vi "Ping.vi"() -> ()   [LabVIEW 2020]
panel:
  in  "Stop":bool
  out "Memory Usage History":sgl(graph)
  out "Memory Usage":sgl
  out "error out":errorcluster
  in  "stop":bool
  out "CPU Usage (%)":sgl(slide) scale=0.0..100.0
  out "Processor History":sgl(graph)
  out "cpu usage":sgl
  out "System Status":string
  in  "STOP VI":bool
  in  "PING IP":bool
  out "IP Free?":bool
  in  "IP Address to Ping":string="0.0.0.0"
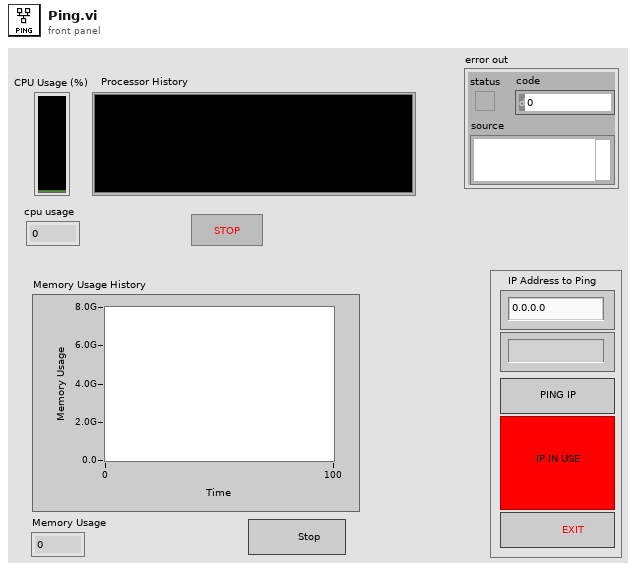
[diagram p1: front panel]
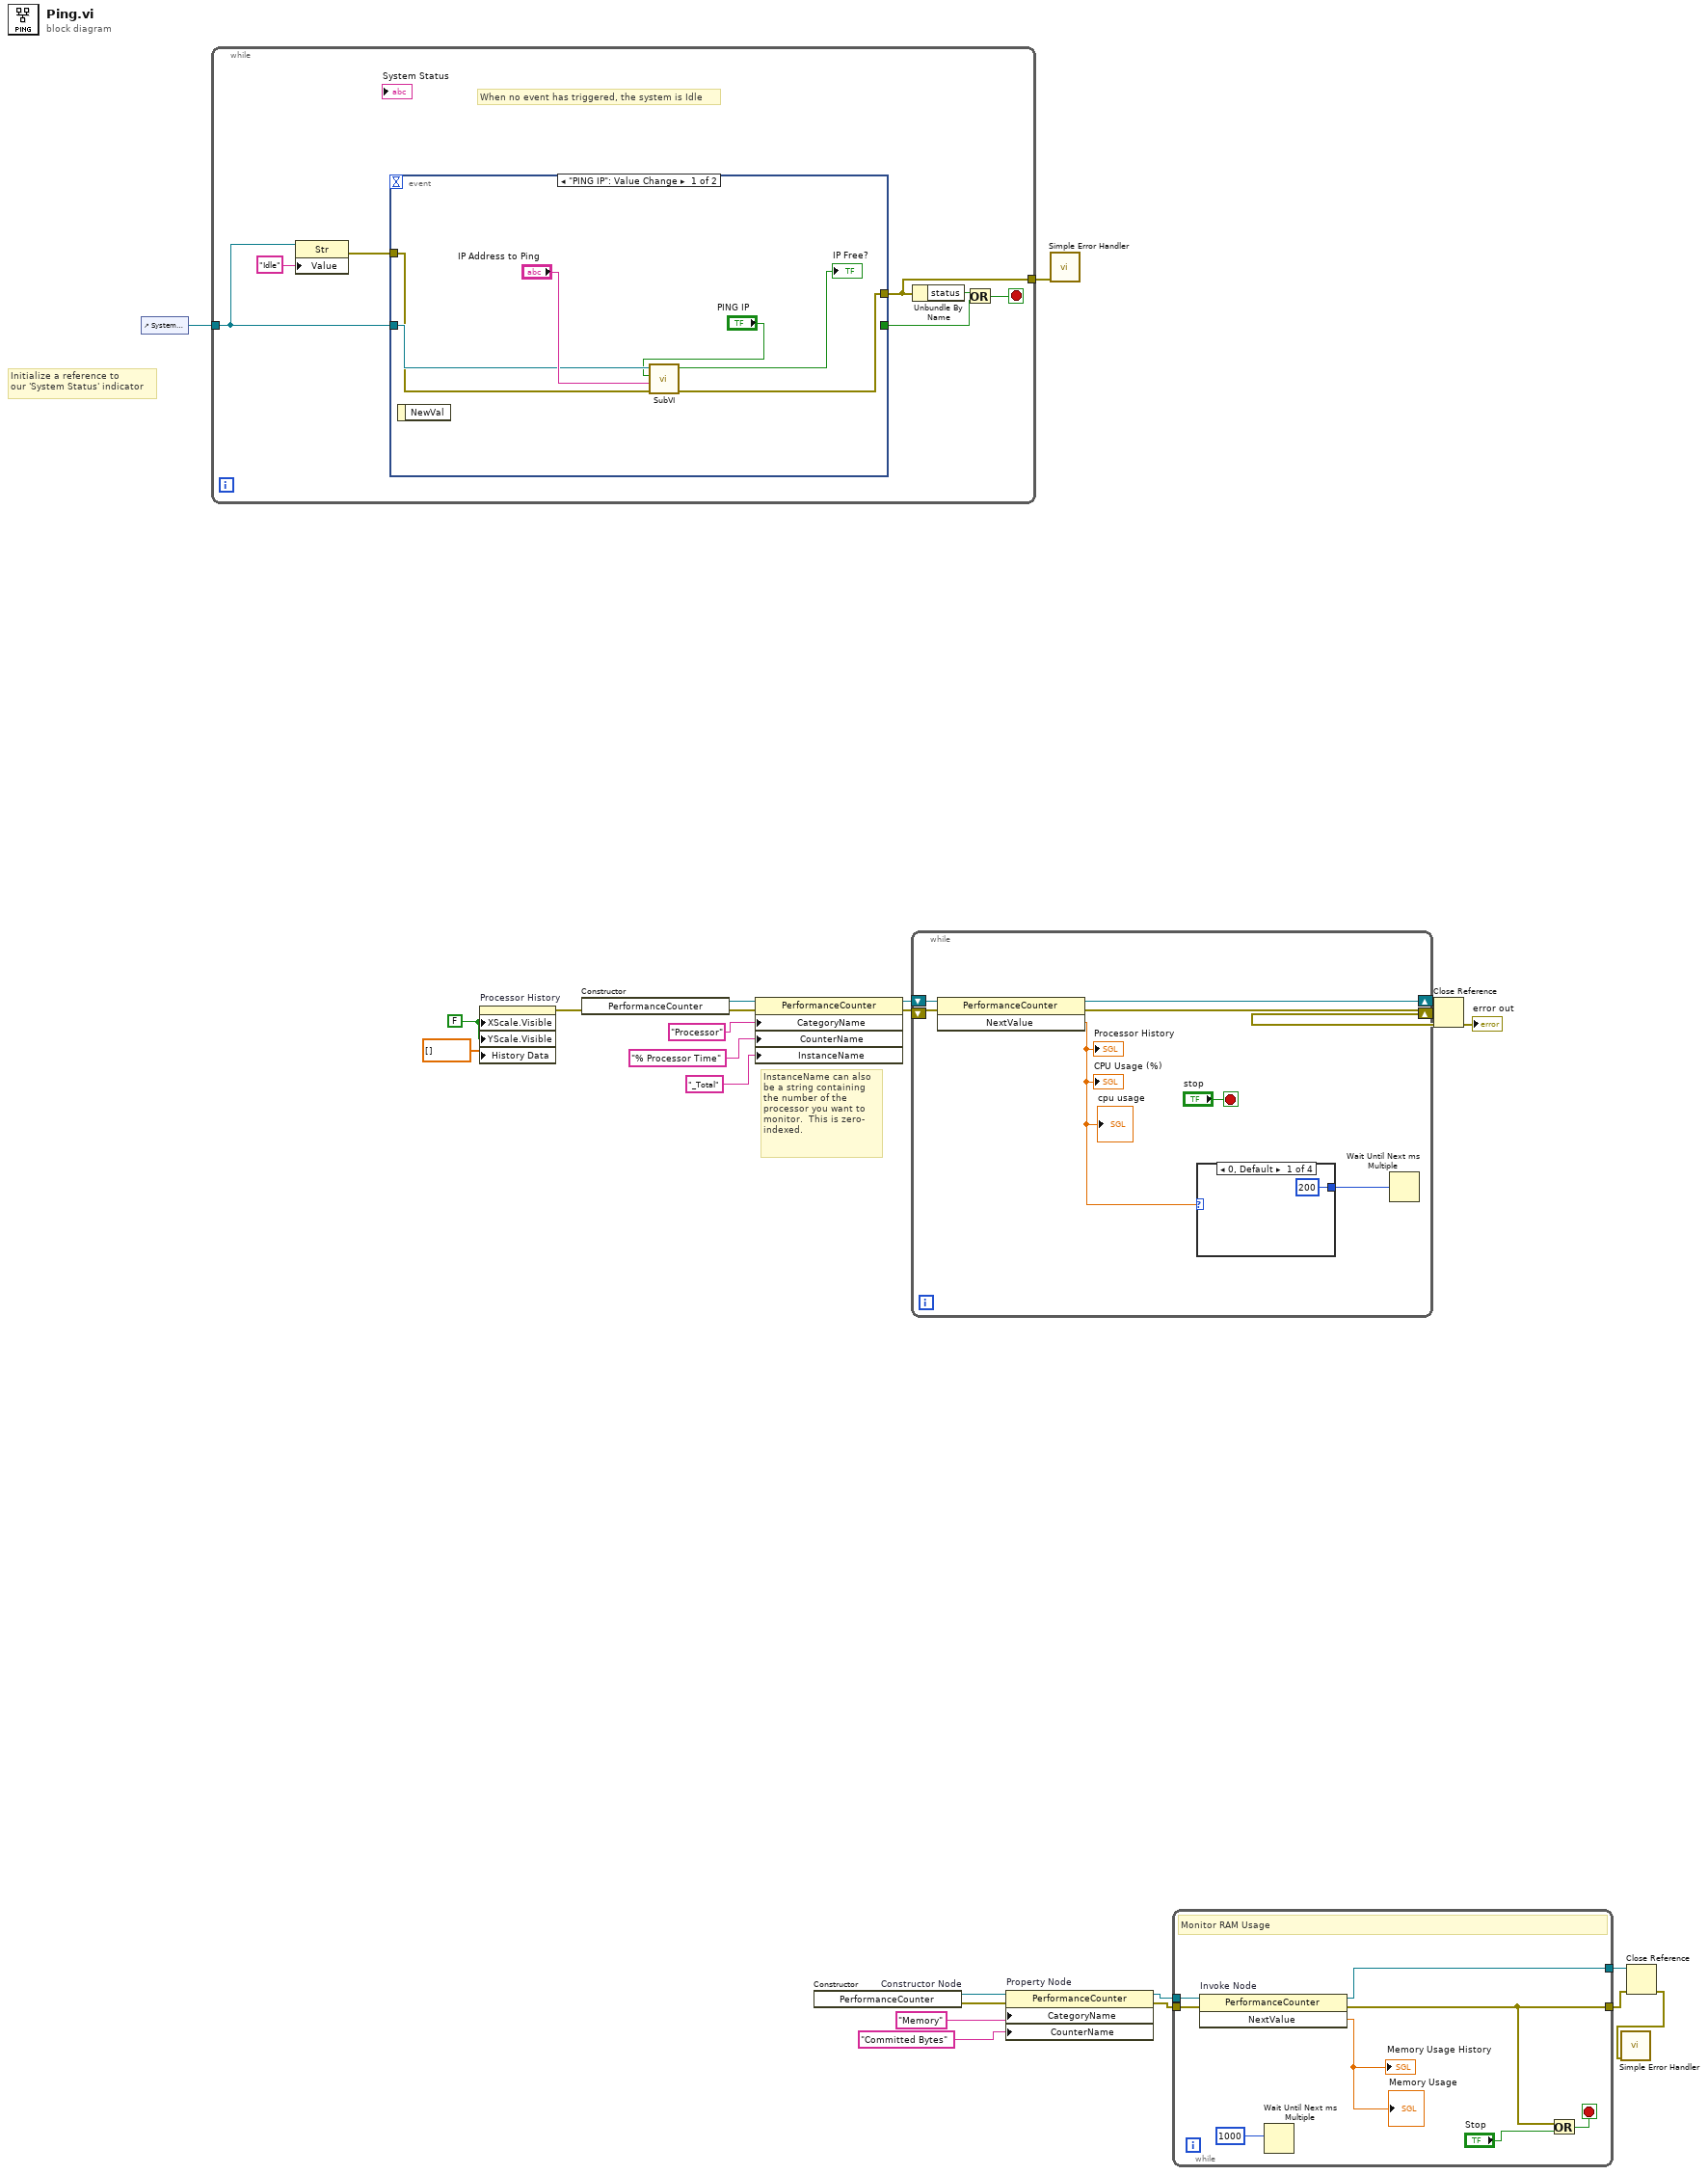
[diagram p0: block diagram]
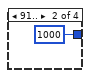
[diagram p2: hidden frame]
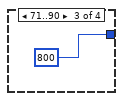
[diagram p3: hidden frame]
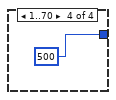
[diagram p4: hidden frame]
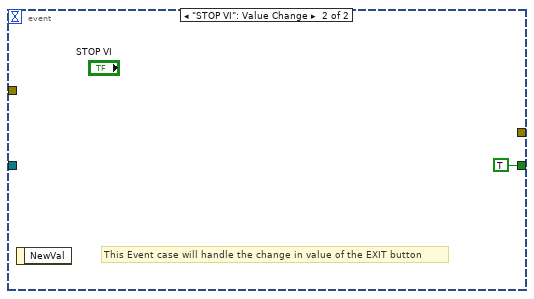
[diagram p5: hidden frame]
diagram:
  w13 = FALSE ("X Scale.Visible")
  # "InstanceName can also\nbe a string containing\nthe number of the\nprocessor you want to\nmonitor.  This is zero-\nindexed."
  # "Initialize a reference to\nour 'System Status' indicator"
  n1 = control-ref of="System Status"() -> (w23:refnum<vi>)
  n2 = while {
    tunnel: [w31] -> w24
    tunnel: w23 -> [w27]
    stop <- w26 stop-if-true
    # "When no event has triggered, the system is Idle"
    n3 = property class="Str"(reference=w27, "Value"="Idle" ("System Status")) -> (error out=w25:errorcluster)  [unwired: 1 in, 1 out]
    n4 = event shown="[0] \"PING IP\": Value Change" {
      selector: _ -> [_ _]
      dyn-events: _ -> [_ _]
      timeout: _ -> [_ _]
      tunnel: [w37 _] -> w31
      tunnel: [_ TRUE] -> w29
      tunnel: w27 -> [w35 _]
      tunnel: w25 -> [w34 _]
      event "PING IP": Value Change {
        n5 = event-data() -> ()  [unwired: 1 in, 1 out]
        n6 = call "SubVI.vi"("error in (no error)"=w34, "IP Address to Ping"="IP Address to Ping", "PING IP"="PING IP", "String in"=w35) -> ("error out"=w37:errorcluster, "IP Free?"=→"IP Free?":bool)  [unwired: 6 in]
      }
      event "STOP VI": Value Change {
        # "This Event case will handle the change in value of the EXIT button"
        n7 = event-data() -> ()  [unwired: 1 in, 1 out]
      }
    }
    n8 = Unbundle By Name(w31) -> ("status"=w30:bool)
    n9 = Or(x=w30, y=w29) -> (x .or. y?=w26:bool)
  }
  n10 = property on="Processor History" class="WFChart (strict)"("XScale.Visible"=w13, "YScale.Visible"=w13, "History Data"=sgl[] []) -> (error out=w10:errorcluster)  [unwired: 2 in, 1 out]
  n11 = constructor class="PerformanceCounter" ("Constructor Node")(error in=w10) -> (reference out=w22:refnum<k24>, error out=w21:errorcluster)  [unwired: 2 in, 1 out]
  n12 = property on="Property Node" class="PerformanceCounter"(reference=w22, error in=w21, "CategoryName"="Processor", "CounterName"="% Processor Time", "InstanceName"="_Total") -> (reference out=w18:refnum<k24>, error out=w17:errorcluster)
  n13 = constructor on="Constructor Node" class="PerformanceCounter"() -> (reference out=w6:refnum<k24>, error out=w5:errorcluster)  [unwired: 3 in, 1 out]
  n14 = while {
    shift-right: [w42] -> w15
    shift-left: w18 -> [w45]
    shift-right: [w43] -> w16
    shift-left: w17 -> [w44]
    stop <- "stop" stop-if-true
    n15 = invoke on="Invoke Node" class="PerformanceCounter" method="NextValue"(reference=w45, error in=w44) -> (reference out=w42:refnum<k24>, error out=w43:errorcluster, "NextValue"=w40:sgl)  [unwired: 1 in]
    "CPU Usage (%)" <- w40
    "Processor History" <- w40
    "cpu usage" <- w40
    n16 = case shown="0, Default" w40 {
      tunnel: [u32 200 ("milliseconds to wait") u32 1000 ("milliseconds to wait") u32 800 ("milliseconds to wait") u32 500 ("milliseconds to wait")] -> w39
      frame 0, Default {
      }
      frame 91.. {
      }
      frame 71..90 {
      }
      frame 1..70 {
      }
    }
    n17 = Wait Until Next ms Multiple(millisecond multiple=w39) -> ()  [unwired: 1 out]
  }
  n18 = property on="Property Node" class="PerformanceCounter"(reference=w6, error in=w5, "CategoryName"="Memory" ("categoryName"), "CounterName"="Committed Bytes" ("counterName")) -> (reference out=w4:refnum<k24>, error out=w3:errorcluster)
  n19 = call <vilib>:"Simple Error Handler.vi"("error in (no error)"=w24) -> ()  [unwired: 4 in, 5 out]
  n20 = while {
    tunnel: w4 -> [w55]
    tunnel: w3 -> [w54]
    tunnel: [w53] -> w9
    tunnel: [w52] -> w7
    stop <- w56 stop-if-true
    # "Monitor RAM Usage"
    n21 = invoke on="Invoke Node" class="PerformanceCounter" method="NextValue"(reference=w55, error in=w54) -> (reference out=w52:refnum<k24>, error out=w53:errorcluster, "NextValue"=→"Memory Usage History" →"Memory Usage":sgl)  [unwired: 1 in]
    n22 = Wait Until Next ms Multiple(millisecond multiple=u32 1000) -> ()  [unwired: 1 out]
    n23 = Or(x=w53, y="Stop") -> (x .or. y?=w56:bool)
  }
  n24 = Close Reference(reference=w15, error in (no error)=w16) -> (error out=→"error out":errorcluster)
  n25 = Close Reference(reference=w7, error in (no error)=w9) -> (error out=w8:errorcluster)
  n26 = call <vilib>:"Simple Error Handler.vi"("error in (no error)"=w8) -> ()  [unwired: 1 in, 8 out]
